vi "Format CSV.vi"(8 "error in (no error)":errorcluster, 9 "delimiter":string=",", 10 "CSV File Input":path, 11 "Original CSV Format":enum16{"Format A", "Format B"}(ring)) -> (0 "error out":errorcluster, 1 "Parcel Length":i32[](array[numeric]), 2 "All Terminal Data":T1(array[cluster]))   [LabVIEW 2017] (continued)
"32:42.2", "32:42.2", "32:42.3", "32:42.3", "32:42.3", "32:42.4", "32:42.4", "32:42.4", "32:42.5", "32:42.5", "32:42.5", "32:42.6", "32:42.6", "32:42.6", "32:42.7", "32:42.7", "32:42.7", "32:42.8", "32:42.8", "32:42.8", "32:42.9", "32:42.9", "32:42.9", "32:43.0", "32:43.0", "32:43.0", "32:43.1", "32:43.1", "32:43.1", "32:43.2", "32:43.2", "32:43.2", "32:43.3", "32:43.3", "32:43.3", "32:43.4", "32:43.4", "32:43.4", "32:43.5", "32:43.5", "32:43.5", "32:43.6", "32:43.6", "32:43.6", "32:43.7", "32:43.7", "32:43.7", "32:43.8", "32:43.8", "32:43.8", "32:43.9", "32:43.9", "32:43.9", "32:44.0", "32:44.0", "32:44.0", "32:44.1", "32:44.1", "32:44.1", "32:44.2", "32:44.2", "32:44.2", "32:44.3", "32:44.3", "32:44.3", "32:44.4", "32:44.4", "32:44.4", "32:44.5", "32:44.5", "32:44.5", "32:44.6", "32:44.6", "32:44.6", "32:44.7", "32:44.7", "32:44.7", "32:44.8", "32:44.8", "32:44.8", "32:44.9", "32:44.9", "32:44.9", "32:45.0", "32:45.0", "32:45.0", "32:45.1", "32:45.1", "32:45.1", "32:45.2", "32:45.2", "32:45.2", "32:45.3", "32:45.3", "32:45.3", "32:45.4", "32:45.4", "32:45.4", "32:45.5", "32:45.5", "32:45.5", "32:45.6", "32:45.6", "32:45.6", "32:45.7", "32:45.7", "32:45.7", "32:45.8", "32:45.8", "32:45.8", "32:45.9", "32:45.9", "32:45.9", "32:46.0", "32:46.0", "32:46.0", "32:46.1", "32:46.1", "32:46.1", "32:46.2", "32:46.2", "32:46.2", "32:46.3", "32:46.3", "32:46.3", "32:46.4", "32:46.4", "32:46.4", "32:46.5", "32:46.5", "32:46.5", "32:46.6", "32:46.6", "32:46.6", "32:46.7", "32:46.7", "32:46.7", "32:46.8", "32:46.8", "32:46.8", "32:46.9", "32:46.9", "32:46.9", "32:47.0", "32:47.0", "32:47.0", "32:47.1", "32:47.1", "32:47.1", "32:47.2", "32:47.2", "32:47.2", "32:47.3", "32:47.3", "32:47.3", "32:47.4", "32:47.4", "32:47.4", "32:47.5", "32:47.5", "32:47.5", "32:47.6", "32:47.6", "32:47.6", "32:47.7", "32:47.7", "32:47.7", "32:47.8", "32:47.8", "32:47.8", "32:47.9", "32:47.9", "32:47.9", "32:48.0", "32:48.0", "32:48.0", "32:48.1", "32:48.1", "32:48.1", "32:48.2", "32:48.2", "32:48.2", "32:48.3", "32:48.3", "32:48.3", "32:48.4", "32:48.4", "32:48.4", "32:48.5", "32:48.5", "32:48.5", "32:48.6", "32:48.6", "32:48.6", "32:48.7", "32:48.7", "32:48.7", "32:48.8", "32:48.8", "32:48.8", "32:48.9", "32:48.9", "32:48.9", "32:49.0", "32:49.0", "32:49.0", "32:49.1", "32:49.1", "32:49.1", "32:49.2", "32:49.2", "32:49.2", "32:49.3", "32:49.3", "32:49.3", "32:49.4", "32:49.4", "32:49.4", "32:49.5", "32:49.5", "32:49.5", "32:49.6", "32:49.6", "32:49.6", "32:49.7", "32:49.7", "32:49.7", "32:49.8", "32:49.8", "32:49.8", "32:49.9", "32:49.9", "32:49.9", "32:50.0", "32:50.0", "32:50.0", "32:50.1", "32:50.1", "32:50.1", "32:50.2", "32:50.2", "32:50.2", "32:50.3", "32:50.3", "32:50.3", "32:50.4", "32:50.4", "32:50.4", "32:50.5", "32:50.5", "32:50.5", "32:50.6", "32:50.6", "32:50.6", "32:50.7", "32:50.7", "32:50.7", "32:50.8", "32:50.8", "32:50.8", "32:50.9", "32:50.9", "32:50.9", "32:51.0", "32:51.0", "32:51.0", "32:51.1", "32:51.1", "32:51.1", "32:51.2", "32:51.2", "32:51.2", "32:51.3", "32:51.3", "32:51.3", "32:51.4", "32:51.4", "32:51.4", "32:51.5", "32:51.5", "32:51.5", "32:51.6", "32:51.6", "32:51.6", "32:51.7", "32:51.7", "32:51.7", "32:51.8", "32:51.8", "32:51.8", "32:51.9", "32:51.9", "32:51.9", "32:52.0", "32:52.0", "32:52.0", "32:52.1", "32:52.1", "32:52.1", "32:52.2", "32:52.2", "32:52.2", "32:52.3", "32:52.3", "32:52.3", "32:52.4", "32:52.4", "32:52.4", "32:52.5", "32:52.5", "32:52.5", "32:52.6", "32:52.6", "32:52.6", "32:52.7", "32:52.7", "32:52.7", "32:52.8", "32:52.8", "32:52.8", "32:52.9", "32:52.9", "32:52.9", "32:53.0", "32:53.0", "32:53.0", "32:53.1", "32:53.1", "32:53.1", "32:53.2", "32:53.2", "32:53.2", "32:53.3", "32:53.3", "32:53.3", "32:53.4", "32:53.4", "32:53.4", "32:53.5", "32:53.5", "32:53.5", "32:53.6", "32:53.6", "32:53.6", "32:53.7", "32:53.7", "32:53.7", "32:53.8", "32:53.8", "32:53.8", "32:53.9", "32:53.9", "32:53.9", "32:54.0", "32:54.0", "32:54.0", "32:54.1", "32:54.1", "32:54.1", "32:54.2", "32:54.2", "32:54.2", "32:54.3", "32:54.3", "32:54.3", "32:54.4", "32:54.4", "32:54.4", "32:54.5", "32:54.5", "32:54.5", "32:54.6", "32:54.6", "32:54.6", "32:54.7", "32:54.7", "32:54.7", "32:54.8", "32:54.8", "32:54.8", "32:54.9", "32:54.9", "32:54.9", "32:55.0", "32:55.0", "32:55.0", "32:55.1", "32:55.1", "32:55.1", "32:55.2", "32:55.2", "32:55.2", "32:55.3", "32:55.3", "32:55.3", "32:55.4", "32:55.4", "32:55.4", "32:55.5", "32:55.5", "32:55.5", "32:55.6", "32:55.6", "32:55.6", "32:55.7", "32:55.7", "32:55.7", "32:55.8", "32:55.8", "32:55.8", "32:55.9", "32:55.9", "32:55.9", "32:56.0", "32:56.0", "32:56.0", "32:56.1", "32:56.1", "32:56.1", "32:56.2", "32:56.2", "32:56.2", "32:56.3", "32:56.3", "32:56.3", "32:56.4", "32:56.4", "32:56.4", "32:56.5", "32:56.5", "32:56.5", "32:56.6", "32:56.6", "32:56.6", "32:56.7", "32:56.7", "32:56.7", "32:56.8", "32:56.8", "32:56.8", "32:56.9", "32:56.9", "32:56.9", "32:57.0", "32:57.0", "32:57.0", "32:57.1", "32:57.1", "32:57.1", "32:57.2", "32:57.2", "32:57.2", "32:57.3", "32:57.3", "32:57.3", "32:57.4", "32:57.4", "32:57.4", "32:57.5", "32:57.5", "32:57.5", "32:57.6", "32:57.6", "32:57.6", "32:57.7", "32:57.7", "32:57.7", "32:57.8", "32:57.8", "32:57.8", "32:57.9", "32:57.9", "32:57.9", "32:58.0", "32:58.0", "32:58.0", "32:58.1", "32:58.1", "32:58.1", "32:58.2", "32:58.2", "32:58.2", "32:58.3", "32:58.3", "32:58.3", "32:58.4", "32:58.4", "32:58.4", "32:58.5", "32:58.5", "32:58.5", "32:58.6", "32:58.6", "32:58.6", "32:58.7", "32:58.7", "32:58.7", "32:58.8", "32:58.8", "32:58.8", "32:58.9", "32:58.9", "32:58.9", "32:59.0", "32:59.0", "32:59.0", "32:59.1", "32:59.1", "32:59.1", "32:59.2", "32:59.2", "32:59.2", "32:59.3", "32:59.3", "32:59.3", "32:59.4", "32:59.4", "32:59.4", "32:59.5", "32:59.5", "32:59.5", "32:59.6", "32:59.6", "32:59.6", "32:59.7", "32:59.7", "32:59.7", "32:59.8", "32:59.8", "32:59.8", "32:59.9", "32:59.9", "32:59.9", "33:00.0", "33:00.0", "33:00.0", "33:00.1", "33:00.1", "33:00.1", "33:00.2", "33:00.2", "33:00.2", "33:00.3", "33:00.3", "33:00.3", "33:00.4", "33:00.4", "33:00.4", "33:00.5", "33:00.5", "33:00.5", "33:00.6", "33:00.6", "33:00.6", "33:00.7", "33:00.7", "33:00.7", "33:00.8", "33:00.8", "33:00.8", "33:00.9", "33:00.9", "33:00.9", "33:01.0", "33:01.0", "33:01.0", "33:01.1", "33:01.1", "33:01.1", "33:01.2", "33:01.2", "33:01.2", "33:01.3", "33:01.3", "33:01.3", "33:01.4", "33:01.4", "33:01.4", "33:01.5", "33:01.5", "33:01.5", "33:01.6", "33:01.6", "33:01.6", "33:01.7", "33:01.7", "33:01.7", "33:01.8", "33:01.8", "33:01.8", "33:01.9", "33:01.9", "33:01.9", "33:02.0", "33:02.0", "33:02.0", "33:02.1", "33:02.1", "33:02.1", "33:02.2", "33:02.2", "33:02.2", "33:02.3", "33:02.3", "33:02.3", "33:02.4", "33:02.4", "33:02.4", "33:02.5", "33:02.5", "33:02.5", "33:02.6", "33:02.6", "33:02.6", "33:02.7", "33:02.7", "33:02.7", "33:02.8", "33:02.8", "33:02.8", "33:02.9", "33:02.9", "33:02.9", "33:03.0", "33:03.0", "33:03.0", "33:03.1", "33:03.1", "33:03.1", "33:03.2", "33:03.2", "33:03.2", "33:03.3", "33:03.3", "33:03.3", "33:03.4", "33:03.4", "33:03.4", "33:03.5", "33:03.5", "33:03.5", "33:03.6", "33:03.6", "33:03.6", "33:03.7", "33:03.7", "33:03.7", "33:03.8", "33:03.8", "33:03.8", "33:03.9", "33:03.9", "33:03.9", "33:04.0", "33:04.0", "33:04.0", "33:04.1", "33:04.1", "33:04.1", "33:04.2", "33:04.2", "33:04.2", "33:04.3", "33:04.3", "33:04.3", "33:04.4", "33:04.4", "33:04.4", "33:04.5", "33:04.5", "33:04.5", "33:04.6", "33:04.6", "33:04.6", "33:04.7", "33:04.7", "33:04.7", "33:04.8", "33:04.8", "33:04.8", "33:04.9", "33:04.9", "33:04.9", "33:05.0", "33:05.0", "33:05.0", "33:05.1", "33:05.1", "33:05.1", "33:05.2", "33:05.2", "33:05.2", "33:05.3", "33:05.3", "33:05.3", "33:05.4", "33:05.4", "33:05.4", "33:05.5", "33:05.5", "33:05.5", "33:05.6", "33:05.6", "33:05.6", "33:05.7", "33:05.7", "33:05.7", "33:05.8", "33:05.8", "33:05.8", "33:05.9", "33:05.9", "33:05.9", "33:06.0", "33:06.0", "33:06.0", "33:06.1", "33:06.1", "33:06.1", "33:06.2", "33:06.2", "33:06.2", "33:06.3", "33:06.3", "33:06.3", "33:06.4", "33:06.4", "33:06.4", "33:06.5", "33:06.5", "33:06.5", "33:06.6", "33:06.6", "33:06.6", "33:06.7", "33:06.7", "33:06.7", "33:06.8", "33:06.8", "33:06.8", "33:06.9", "33:06.9", "33:06.9", "33:07.0", "33:07.0", "33:07.0", "33:07.1", "33:07.1", "33:07.1", "33:07.2", "33:07.2", "33:07.2", "33:07.3", "33:07.3", "33:07.3", "33:07.4", "33:07.4", "33:07.4", "33:07.5", "33:07.5", "33:07.5", "33:07.6", "33:07.6", "33:07.6", "33:07.7", "33:07.7", "33:07.7", "33:07.8", "33:07.8", "33:07.8", "33:07.9", "33:07.9", "33:07.9", "33:08.0", "33:08.0", "33:08.0", "33:08.1", "33:08.1", "33:08.1", "33:08.2", "33:08.2", "33:08.2", "33:08.3", "33:08.3", "33:08.3", "33:08.4", "33:08.4", "33:08.4", "33:08.5", "33:08.5", "33:08.5", "33:08.6", "33:08.6", "33:08.6", "33:08.7", "33:08.7", "33:08.7", "33:08.8", "33:08.8", "33:08.8", "33:08.9", "33:08.9", "33:08.9", "33:09.0", "33:09.0", "33:09.0", "33:09.1", "33:09.1", "33:09.1", "33:09.2", "33:09.2", "33:09.2", "33:09.3", "33:09.3", "33:09.3", "33:09.4", "33:09.4", "33:09.4", "33:09.5", "33:09.5", "33:09.5", "33:09.6", "33:09.6", "33:09.6", "33:09.7", "33:09.7", "33:09.7", "33:09.8", "33:09.8", "33:09.8", "33:09.9", "33:09.9", "33:09.9", "33:10.0", "33:10.0", "33:10.0", "33:10.1", "33:10.1", "33:10.1", "33:10.2", "33:10.2", "33:10.2", "33:10.3", "33:10.3", "33:10.3", "33:10.4", "33:10.4", "33:10.4", "33:10.5", "33:10.5", "33:10.5", "33:10.6", "33:10.6", "33:10.6", "33:10.7", "33:10.7", "33:10.7", "33:10.8", "33:10.8", "33:10.8", "33:10.9", "33:10.9", "33:10.9", "33:11.0", "33:11.0", "33:11.0", "33:11.1", "33:11.1", "33:11.1", "33:11.2", "33:11.2", "33:11.2", "33:11.3", "33:11.3", "33:11.3", "33:11.4", "33:11.4", "33:11.4", "33:11.5", "33:11.5", "33:11.5", "33:11.6", "33:11.6", "33:11.6", "33:11.7", "33:11.7", "33:11.7", "33:11.8", "33:11.8", "33:11.8", "33:11.9", "33:11.9", "33:11.9", "33:12.0", "33:12.0", "33:12.0", "33:12.1", "33:12.1", "33:12.1", "33:12.2", "33:12.2", "33:12.2", "33:12.3", "33:12.3", "33:12.3", "33:12.4", "33:12.4", "33:12.4", "33:12.5", "33:12.5", "33:12.5", "33:12.6", "33:12.6", "33:12.6", "33:12.7", "33:12.7", "33:12.7", "33:12.8", "33:12.8", "33:12.8", "33:12.9", "33:12.9", "33:12.9", "33:13.0", "33:13.0", "33:13.0", "33:13.1", "33:13.1", "33:13.1", "33:13.2", "33:13.2", "33:13.2", "33:13.3", "33:13.3", "33:13.3", "33:13.4", "33:13.4", "33:13.4", "33:13.5", "33:13.5", "33:13.5", "33:13.6", "33:13.6", "33:13.6", "33:13.7", "33:13.7", "33:13.7", "33:13.8", "33:13.8", "33:13.8", "33:13.9", "33:13.9", "33:13.9", "33:14.0", "33:14.0", "33:14.0", "33:14.1", "33:14.1", "33:14.1", "33:14.2", "33:14.2", "33:14.2", "33:14.3", "33:14.3", "33:14.3", "33:14.4", "33:14.4", "33:14.4", "33:14.5", "33:14.5", "33:14.5", "33:14.6", "33:14.6", "33:14.6", "33:14.7", "33:14.7", "33:14.7", "33:14.8", "33:14.8", "33:14.8", "33:14.9", "33:14.9", "33:14.9", "33:15.0", "33:15.0", "33:15.0", "33:15.1", "33:15.1", "33:15.1", "33:15.2", "33:15.2", "33:15.2", "33:15.3", "33:15.3", "33:15.3", "33:15.4", "33:15.4", "33:15.4", "33:15.5", "33:15.5", "33:15.5", "33:15.6", "33:15.6", "33:15.6", "33:15.7", "33:15.7", "33:15.7", "33:15.8", "33:15.8", "33:15.8", "33:15.9", "33:15.9", "33:15.9", "33:16.0", "33:16.0", "33:16.0", "33:16.1", "33:16.1", "33:16.1", "33:16.2", "33:16.2", "33:16.2", "33:16.3", "33:16.3", "33:16.3", "33:16.4", "33:16.4", "33:16.4", "33:16.5", "33:16.5", "33:16.5", "33:16.6", "33:16.6", "33:16.6", "33:16.7", "33:16.7", "33:16.7", "33:16.8", "33:16.8", "33:16.8", "33:16.9", "33:16.9", "33:16.9", "33:17.0", "33:17.0", "33:17.0", "33:17.1", "33:17.1", "33:17.1", "33:17.2", "33:17.2", "33:17.2", "33:17.3", "33:17.3", "33:17.3", "33:17.4", "33:17.4", "33:17.4", "33:17.5", "33:17.5", "33:17.5", "33:17.6", "33:17.6", "33:17.6", "33:17.7", "33:17.7", "33:17.7", "33:17.8", "33:17.8", "33:17.8", "33:17.9", "33:17.9", "33:17.9", "33:18.0", "33:18.0", "33:18.0", "33:18.1", "33:18.1", "33:18.1", "33:18.2", "33:18.2", "33:18.2", "33:18.3", "33:18.3", "33:18.3", "33:18.4", "33:18.4", "33:18.4", "33:18.5", "33:18.5", "33:18.5", "33:18.6", "33:18.6", "33:18.6", "33:18.7", "33:18.7", "33:18.7", "33:18.8", "33:18.8", "33:18.8", "33:18.9", "33:18.9", "33:18.9", "33:19.0", "33:19.0", "33:19.0", "33:19.1", "33:19.1", "33:19.1", "33:19.2", "33:19.2", "33:19.2", "33:19.3", "33:19.3", "33:19.3", "33:19.4", "33:19.4", "33:19.4", "33:19.5", "33:19.5", "33:19.5", "33:19.6", "33:19.6", "33:19.6", "33:19.7", "33:19.7", "33:19.7", "33:19.8", "33:19.8", "33:19.8", "33:19.9", "33:19.9", "33:19.9", "33:20.0", "33:20.0", "33:20.0", "33:20.1", "33:20.1", "33:20.1", "33:20.2", "33:20.2", "33:20.2", "33:20.3", "33:20.3", "33:20.3", "33:20.4", "33:20.4", "33:20.4", "33:20.5", "33:20.5", "33:20.5", "33:20.6", "33:20.6", "33:20.6", "33:20.7", "33:20.7", "33:20.7", "33:20.8", "33:20.8", "33:20.8", "33:20.9", "33:20.9", "33:20.9", "33:21.0", "33:21.0", "33:21.0", "33:21.1", "33:21.1", "33:21.1", "33:21.2", "33:21.2", "33:21.2", "33:21.3", "33:21.3", "33:21.3", "33:21.4", "33:21.4", "33:21.4", "33:21.5", "33:21.5", "33:21.5", "33:21.6", "33:21.6", "33:21.6", "33:21.7", "33:21.7", "33:21.7", "33:21.8", "33:21.8", "33:21.8", "33:21.9", "33:21.9", "33:21.9", "33:22.0", "33:22.0", "33:22.0", "33:22.1", "33:22.1", "33:22.1", "33:22.2", "33:22.2", "33:22.2", "33:22.3", "33:22.3", "33:22.3", "33:22.4", "33:22.4", "33:22.4", "33:22.5", "33:22.5", "33:22.5", "33:22.6", "33:22.6", "33:22.6", "33:22.7", "33:22.7", "33:22.7", "33:22.8", "33:22.8", "33:22.8", "33:22.9", "33:22.9", "33:22.9", "33:23.0", "33:23.0", "33:23.0", "33:23.1", "33:23.1", "33:23.1", "33:23.2", "33:23.2", "33:23.2", "33:23.3", "33:23.3", "33:23.3", "33:23.4", "33:23.4", "33:23.4", "33:23.5", "33:23.5", "33:23.5", "33:23.6", "33:23.6", "33:23.6", "33:23.7", "33:23.7", "33:23.7", "33:23.8", "33:23.8", "33:23.8", "33:23.9", "33:23.9", "33:23.9", "33:24.0", "33:24.0", "33:24.0", "33:24.1", "33:24.1", "33:24.1", "33:24.2", "33:24.2", "33:24.2", "33:24.3", "33:24.3", "33:24.3", "33:24.4", "33:24.4", "33:24.4", "33:24.5", "33:24.5", "33:24.5", "33:24.6", "33:24.6", "33:24.6", "33:24.7", "33:24.7", "33:24.7", "33:24.8", "33:24.8", "33:24.8", "33:24.9", "33:24.9", "33:24.9", "33:25.0", "33:25.0", "33:25.0", "33:25.1", "33:25.1", "33:25.1", "33:25.2", "33:25.2", "33:25.2", "33:25.3", "33:25.3", "33:25.3", "33:25.4", "33:25.4", "33:25.4", "33:25.5", "33:25.5", "33:25.5", "33:25.6", "33:25.6", "33:25.6", "33:25.7", "33:25.7", "33:25.7", "33:25.8", "33:25.8", "33:25.8", "33:25.9", "33:25.9", "33:25.9", "33:26.0", "33:26.0", "33:26.0", "33:26.1", "33:26.1", "33:26.1", "33:26.2", "33:26.2", "33:26.2", "33:26.3", "33:26.3", "33:26.3", "33:26.4", "33:26.4", "33:26.4", "33:26.5", "33:26.5", "33:26.5", "33:26.6", "33:26.6", "33:26.6", "33:26.7", "33:26.7", "33:26.7", "33:26.8", "33:26.8", "33:26.8", "33:26.9", "33:26.9", "33:26.9", "33:27.0", "33:27.0", "33:27.0", "33:27.1", "33:27.1", "33:27.1", "33:27.2", "33:27.2", "33:27.2", "33:27.3", "33:27.3", "33:27.3", "33:27.4", "33:27.4", "33:27.4", "33:27.5", "33:27.5", "33:27.5", "33:27.6", "33:27.6", "33:27.6", "33:27.7", "33:27.7", "33:27.7", "33:27.8", "33:27.8", "33:27.8", "33:27.9", "33:27.9", "33:27.9", "33:28.0", "33:28.0", "33:28.0", "33:28.1", "33:28.1", "33:28.1", "33:28.2", "33:28.2", "33:28.2", "33:28.3", "33:28.3", "33:28.3", "33:28.4", "33:28.4", "33:28.4", "33:28.5", "33:28.5", "33:28.5", "33:28.6", "33:28.6", "33:28.6", "33:28.7", "33:28.7", "33:28.7", "33:28.8", "33:28.8", "33:28.8", "33:28.9", "33:28.9", "33:28.9", "33:29.0", "33:29.0", "33:29.0", "33:29.1", "33:29.1", "33:29.1", "33:29.2", "33:29.2", "33:29.2", "33:29.3", "33:29.3", "33:29.3", "33:29.4", "33:29.4", "33:29.4", "33:29.5", "33:29.5", "33:29.5", "33:29.6", "33:29.6", "33:29.6", "33:29.7", "33:29.7", "33:29.7", "33:29.8", "33:29.8", "33:29.8", "33:29.9", "33:29.9", "33:29.9", "33:30.0", "33:30.0", "33:30.0", "33:30.1", "33:30.1", "33:30.1", "33:30.2", "33:30.2", "33:30.2", "33:30.3", "33:30.3", "33:30.3", "33:30.4", "33:30.4", "33:30.4", "33:30.5", "33:30.5", "33:30.5", "33:30.6", "33:30.6", "33:30.6", "33:30.7", "33:30.7", "33:30.7", "33:30.8", "33:30.8", "33:30.8", "33:30.9", "33:30.9", "33:30.9", "33:31.0", "33:31.0", "33:31.0", "33:31.1", "33:31.1", "33:31.1", "33:31.2", "33:31.2", "33:31.2", "33:31.3", "33:31.3", "33:31.3", "33:31.4", "33:31.4", "33:31.4", "33:31.5", "33:31.5", "33:31.5", "33:31.6", "33:31.6", "33:31.6", "33:31.7", "33:31.7", "33:31.7", "33:31.8", "33:31.8", "33:31.8", "33:31.9", "33:31.9", "33:31.9", "33:32.0", "33:32.0", "33:32.0", "33:32.1", "33:32.1", "33:32.1", "33:32.2", "33:32.2", "33:32.2", "33:32.3", "33:32.3", "33:32.3", "33:32.4", "33:32.4", "33:32.4", "33:32.5", "33:32.5", "33:32.5", "33:32.6", "33:32.6", "33:32.6", "33:32.7", "33:32.7", "33:32.7", "33:32.8", "33:32.8", "33:32.8", "33:32.9", "33:32.9", "33:32.9", "33:33.0", "33:33.0", "33:33.0", "33:33.1", "33:33.1", "33:33.1", "33:33.2", "33:33.2", "33:33.2", "33:33.3", "33:33.3", "33:33.3", "33:33.4", "33:33.4", "33:33.4", "33:33.5", "33:33.5", "33:33.5", "33:33.6", "33:33.6", "33:33.6", "33:33.7", "33:33.7", "33:33.7", "33:33.8", "33:33.8", "33:33.8", "33:33.9", "33:33.9", "33:33.9", "33:34.0", "33:34.0", "33:34.0", "33:34.1", "33:34.1", "33:34.1", "33:34.2", "33:34.2", "33:34.2", "33:34.3", "33:34.3", "33:34.3", "33:34.4", "33:34.4", "33:34.4", "33:34.5", "33:34.5", "33:34.5", "33:34.6", "33:34.6", "33:34.6", "33:34.7", "33:34.7", "33:34.7", "33:34.8", "33:34.8", "33:34.8", "33:34.9", "33:34.9", "33:34.9", "33:35.0", "33:35.0", "33:35.0", "33:35.1", "33:35.1", "33:35.1", "33:35.2", "33:35.2", "33:35.2", "33:35.3", "33:35.3", "33:35.3", "33:35.4", "33:35.4", "33:35.4", "33:35.5", "33:35.5", "33:35.5", "33:35.6", "33:35.6", "33:35.6", "33:35.7", "33:35.7", "33:35.7", "33:35.8", "33:35.8", "33:35.8", "33:35.9", "33:35.9", "33:35.9", "33:36.0", "33:36.0", "33:36.0", "33:36.1", "33:36.1", "33:36.1", "33:36.2", "33:36.2", "33:36.2", "33:36.3", "33:36.3", "33:36.3", "33:36.4", "33:36.4", "33:36.4", "33:36.5", "33:36.5", "33:36.5", "33:36.6", "33:36.6", "33:36.6", "33:36.7", "33:36.7", "33:36.7", "33:36.8", "33:36.8", "33:36.8", "33:36.9", "33:36.9", "33:36.9", "33:37.0", "33:37.0", "33:37.0", "33:37.1", "33:37.1", "33:37.1", "33:37.2", "33:37.2", "33:37.2", "33:37.3", "33:37.3", "33:37.3", "33:37.4", "33:37.4", "33:37.4", "33:37.5", "33:37.5", "33:37.5", "33:37.6", "33:37.6", "33:37.6", "33:37.7", "33:37.7", "33:37.7", "33:37.8", "33:37.8", "33:37.8", "33:37.9", "33:37.9", "33:37.9", "33:38.0", "33:38.0", "33:38.0", "33:38.1", "33:38.1", "33:38.1", "33:38.2", "33:38.2", "33:38.2", "33:38.3", "33:38.3", "33:38.3", "33:38.4", "33:38.4", "33:38.4", "33:38.5", "33:38.5", "33:38.5", "33:38.6", "33:38.6", "33:38.6", "33:38.7", "33:38.7", "33:38.7", "33:38.8", "33:38.8", "33:38.8", "33:38.9", "33:38.9", "33:38.9", "33:39.0", "33:39.0", "33:39.0", "33:39.1", "33:39.1", "33:39.1", "33:39.2", "33:39.2", "33:39.2", "33:39.3", "33:39.3", "33:39.3", "33:39.4", "33:39.4", "33:39.4", "33:39.5", "33:39.5", "33:39.5", "33:39.6", "33:39.6", "33:39.6", "33:39.7", "33:39.7", "33:39.7", "33:39.8", "33:39.8", "33:39.8", "33:39.9", "33:39.9", "33:39.9", "33:40.0", "33:40.0", "33:40.0", "33:40.1", "33:40.1", "33:40.1", "33:40.2", "33:40.2", "33:40.2", "33:40.3", "33:40.3", "33:40.3", "33:40.4", "33:40.4", "33:40.4", "33:40.5", "33:40.5", "33:40.5", "33:40.6", "33:40.6", "33:40.6", "33:40.7", "33:40.7", "33:40.7", "33:40.8", "33:40.8", "33:40.8", "33:40.9", "33:40.9", "33:40.9", "33:41.0", "33:41.0", "33:41.0", "33:41.1", "33:41.1", "33:41.1", "33:41.2", "33:41.2", "33:41.2", "33:41.3", "33:41.3", "33:41.3", "33:41.4", "33:41.4", "33:41.4", "33:41.5", "33:41.5", "33:41.5", "33:41.6", "33:41.6", "33:41.6", "33:41.7", "33:41.7", "33:41.7", "33:41.8", "33:41.8", "33:41.8", "33:41.9", "33:41.9", "33:41.9", "33:42.0", "33:42.0", "33:42.0", "33:42.1", "33:42.1", "33:42.1", "33:42.2", "33:42.2", "33:42.2", "33:42.3", "33:42.3", "33:42.3", "33:42.4", "33:42.4", "33:42.4", "33:42.5", "33:42.5", "33:42.5", "33:42.6", "33:42.6", "33:42.6", "33:42.7", "33:42.7", "33:42.7", "33:42.8", "33:42.8", "33:42.8", "33:42.9", "33:42.9", "33:42.9", "33:43.0", "33:43.0", "33:43.0", "33:43.1", "33:43.1", "33:43.1", "33:43.2", "33:43.2", "33:43.2", "33:43.3", "33:43.3", "33:43.3", "33:43.4", "33:43.4", "33:43.4", "33:43.5", "33:43.5", "33:43.5", "33:43.6", "33:43.6", "33:43.6", "33:43.7", "33:43.7", "33:43.7", "33:43.8", "33:43.8", "33:43.8", "33:43.9", "33:43.9", "33:43.9", "33:44.0", "33:44.0", "33:44.0", "33:44.1", "33:44.1", "33:44.1", "33:44.2", "33:44.2", "33:44.2", "33:44.3", "33:44.3", "33:44.3", "33:44.4", "33:44.4", "33:44.4", "33:44.5", "33:44.5", "33:44.5", "33:44.6", "33:44.6", "33:44.6", "33:44.7", "33:44.7", "33:44.7", "33:44.8", "33:44.8", "33:44.8", "33:44.9", "33:44.9", "33:44.9", "33:45.0", "33:45.0", "33:45.0", "33:45.1", "33:45.1", "33:45.1", "33:45.2", "33:45.2", "33:45.2", "33:45.3", "33:45.3", "33:45.3", "33:45.4", "33:45.4", "33:45.4", "33:45.5", "33:45.5", "33:45.5", "33:45.6", "33:45.6", "33:45.6", "33:45.7", "33:45.7", "33:45.7", "33:45.8", "33:45.8", "33:45.8", "33:45.9", "33:45.9", "33:45.9", "33:46.0", "33:46.0", "33:46.0", "33:46.1", "33:46.1", "33:46.1", "33:46.2", "33:46.2", "33:46.2", "33:46.3", "33:46.3", "33:46.3", "33:46.4", "33:46.4", "33:46.4", "33:46.5", "33:46.5", "33:46.5", "33:46.6", "33:46.6", "33:46.6", "33:46.7", "33:46.7", "33:46.7", "33:46.8", "33:46.8", "33:46.8", "33:46.9", "33:46.9", "33:46.9", "33:47.0", "33:47.0", "33:47.0", "33:47.1", "33:47.1", "33:47.1", "33:47.2", "33:47.2", "33:47.2", "33:47.3", "33:47.3", "33:47.3", "33:47.4", "33:47.4", "33:47.4", "33:47.5", "33:47.5", "33:47.5", "33:47.6", "33:47.6", "33:47.6", "33:47.7", "33:47.7", "33:47.7", "33:47.8", "33:47.8", "33:47.8", "33:47.9", "33:47.9", "33:47.9", "33:48.0", "33:48.0", "33:48.0", "33:48.1", "33:48.1", "33:48.1", "33:48.2", "33:48.2", "33:48.2", "33:48.3", "33:48.3", "33:48.3", "33:48.4", "33:48.4", "33:48.4", "33:48.5", "33:48.5", "33:48.5", "33:48.6", "33:48.6", "33:48.6", "33:48.7", "33:48.7", "33:48.7", "33:48.8", "33:48.8", "33:48.8", "33:48.9", "33:48.9", "33:48.9", "33:49.0", "33:49.0", "33:49.0", "33:49.1", "33:49.1", "33:49.1", "33:49.2", "33:49.2", "33:49.2", "33:49.3", "33:49.3", "33:49.3", "33:49.4", "33:49.4", "33:49.4", "33:49.5", "33:49.5", "33:49.5", "33:49.6", "33:49.6", "33:49.6", "33:49.7", "33:49.7", "33:49.7", "33:49.8", "33:49.8", "33:49.8", "33:49.9", "33:49.9", "33:49.9", "33:50.0", "33:50.0", "33:50.0", "33:50.1", "33:50.1", "33:50.1", "33:50.2", "33:50.2", "33:50.2", "33:50.3", "33:50.3", "33:50.3", "33:50.4", "33:50.4", "33:50.4", "33:50.5", "33:50.5", "33:50.5", "33:50.6", "33:50.6", "33:50.6", "33:50.7", "33:50.7", "33:50.7", "33:50.8", "33:50.8", "33:50.8", "33:50.9", "33:50.9", "33:50.9", "33:51.0", "33:51.0", "33:51.0", "33:51.1", "33:51.1", "33:51.1", "33:51.2", "33:51.2", "33:51.2", "33:51.3", "33:51.3", "33:51.3", "33:51.4", "33:51.4", "33:51.4", "33:51.5", "33:51.5", "33:51.5", "33:51.6", "33:51.6", "33:51.6", "33:51.7", "33:51.7", "33:51.7", "33:51.8", "33:51.8", "33:51.8", "33:51.9", "33:51.9", "33:51.9", "33:52.0", "33:52.0", "33:52.0", "33:52.1", "33:52.1", "33:52.1", "33:52.2", "33:52.2", "33:52.2", "33:52.3", "33:52.3", "33:52.3", "33:52.4", "33:52.4", "33:52.4", "33:52.5", "33:52.5", "33:52.5", "33:52.6", "33:52.6", "33:52.6", "33:52.7", "33:52.7", "33:52.7", "33:52.8", "33:52.8", "33:52.8", "33:52.9", "33:52.9", "33:52.9", "33:53.0", "33:53.0", "33:53.0", "33:53.1", "33:53.1", "33:53.1", "33:53.2", "33:53.2", "33:53.2", "33:53.3", "33:53.3", "33:53.3", "33:53.4", "33:53.4", "33:53.4", "33:53.5", "33:53.5", "33:53.5", "33:53.6", "33:53.6", "33:53.6", "33:53.7", "33:53.7", "33:53.7", "33:53.8", "33:53.8", "33:53.8", "33:53.9", "33:53.9", "33:53.9", "33:54.0", "33:54.0", "33:54.0", "33:54.1", "33:54.1", "33:54.1", "33:54.2", "33:54.2", "33:54.2", "33:54.3", "33:54.3", "33:54.3", "33:54.4", "33:54.4", "33:54.4", "33:54.5", "33:54.5", "33:54.5", "33:54.6", "33:54.6", "33:54.6", "33:54.7", "33:54.7", "33:54.7", "33:54.8", "33:54.8", "33:54.8", "33:54.9", "33:54.9", "33:54.9", "33:55.0", "33:55.0", "33:55.0", "33:55.1", "33:55.1", "33:55.1", "33:55.2", "33:55.2", "33:55.2", "33:55.3", "33:55.3", "33:55.3", "33:55.4", "33:55.4", "33:55.4", "33:55.5", "33:55.5", "33:55.5", "33:55.6", "33:55.6", "33:55.6", "33:55.7", "33:55.7", "33:55.7", "33:55.8", "33:55.8", "33:55.8", "33:55.9", "33:55.9", "33:55.9", "33:56.0", "33:56.0", "33:56.0", "33:56.1", "33:56.1", "33:56.1", "33:56.2", "33:56.2", "33:56.2", "33:56.3", "33:56.3", "33:56.3", "33:56.4", "33:56.4", "33:56.4", "33:56.5", "33:56.5", "33:56.5", "33:56.6", "33:56.6", "33:56.6", "33:56.7", "33:56.7", "33:56.7", "33:56.8", "33:56.8", "33:56.8", "33:56.9", "33:56.9", "33:56.9", "33:57.0", "33:57.0", "33:57.0", "33:57.1", "33:57.1", "33:57.1", "33:57.2", "33:57.2", "33:57.2", "33:57.3", "33:57.3", "33:57.3", "33:57.4", "33:57.4", "33:57.4", "33:57.5", "33:57.5", "33:57.5", "33:57.6", "33:57.6", "33:57.6", "33:57.7", "33:57.7", "33:57.7", "33:57.8", "33:57.8", "33:57.8", "33:57.9", "33:57.9", "33:57.9", "33:58.0", "33:58.0", "33:58.0", "33:58.1", "33:58.1", "33:58.1", "33:58.2", "33:58.2", "33:58.2", "33:58.3", "33:58.3", "33:58.3", "33:58.4", "33:58.4", "33:58.4", "33:58.5", "33:58.5", "33:58.5", "33:58.6", "33:58.6", "33:58.6", "33:58.7", "33:58.7", "33:58.7", "33:58.8", "33:58.8", "33:58.8", "33:58.9", "33:58.9", "33:58.9", "33:59.0", "33:59.0", "33:59.0", "33:59.1", "33:59.1", "33:59.1", "33:59.2", "33:59.2", "33:59.2", "33:59.3", "33:59.3", "33:59.3", "33:59.4", "33:59.4", "33:59.4", "33:59.5", "33:59.5", "33:59.5", "33:59.6", "33:59.6", "33:59.6", "33:59.7", "33:59.7", "33:59.7", "33:59.8", "33:59.8", "33:59.8", "33:59.9", "33:59.9", "33:59.9", "34:00.0", "34:00.0", "34:00.0", "34:00.1", "34:00.1", "34:00.1", "34:00.2", "34:00.2", "34:00.2", "34:00.3", "34:00.3", "34:00.3", "34:00.4", "34:00.4", "34:00.4", "34:00.5", "34:00.5", "34:00.5", "34:00.6", "34:00.6", "34:00.6", "34:00.7", "34:00.7", "34:00.7", "34:00.8", "34:00.8", "34:00.8", "34:00.9", "34:00.9", "34:00.9", "34:01.0", "34:01.0", "34:01.0", "34:01.1", "34:01.1", "34:01.1", "34:01.2", "34:01.2", "34:01.2", "34:01.3", "34:01.3", "34:01.3", "34:01.4", "34:01.4", "34:01.4", "34:01.5", "34:01.5", "34:01.5", "34:01.6", "34:01.6", "34:01.6", "34:01.7", "34:01.7", "34:01.7", "34:01.8", "34:01.8", "34:01.8", "34:01.9", "34:01.9", "34:01.9", "34:02.0", "34:02.0", "34:02.0", "34:02.1", "34:02.1", "34:02.1", "34:02.2", "34:02.2", "34:02.2", "34:02.3", "34:02.3", "34:02.3", "34:02.4", "34:02.4", "34:02.4", "34:02.5", "34:02.5", "34:02.5", "34:02.6", "34:02.6", "34:02.6", "34:02.7", "34:02.7", "34:02.7", "34:02.8", "34:02.8", "34:02.8", "34:02.9", "34:02.9", "34:02.9", "34:03.0", "34:03.0", "34:03.0", "34:03.1", "34:03.1", "34:03.1", "34:03.2", "34:03.2", "34:03.2", "34:03.3", "34:03.3", "34:03.3", "34:03.4", "34:03.4", "34:03.4", "34:03.5", "34:03.5", "34:03.5", "34:03.6", "34:03.6", "34:03.6", "34:03.7", "34:03.7", "34:03.7", "34:03.8", "34:03.8", "34:03.8", "34:03.9", "34:03.9", "34:03.9", "34:04.0", "34:04.0", "34:04.0", "34:04.1", "34:04.1", "34:04.1", "34:04.2", "34:04.2", "34:04.2", "34:04.3", "34:04.3", "34:04.3", "34:04.4", "34:04.4", "34:04.4", "34:04.5", "34:04.5", "34:04.5", "34:04.6", "34:04.6", "34:04.6", "34:04.7", "34:04.7", "34:04.7", "34:04.8", "34:04.8", "34:04.8", "34:04.9", "34:04.9", "34:04.9", "34:05.0", "34:05.0", "34:05.0", "34:05.1", "34:05.1", "34:05.1", "34:05.2", "34:05.2", "34:05.2", "34:05.3", "34:05.3", "34:05.3", "34:05.4", "34:05.4", "34:05.4", "34:05.5", "34:05.5", "34:05.5", "34:05.6", "34:05.6", "34:05.6", "34:05.7", "34:05.7", "34:05.7", "34:05.8", "34:05.8", "34:05.8", "34:05.9", "34:05.9", "34:05.9", "34:06.0", "34:06.0", "34:06.0", "34:06.1", "34:06.1", "34:06.1", "34:06.2", "34:06.2", "34:06.2", "34:06.3", "34:06.3", "34:06.3", "34:06.4", "34:06.4", "34:06.4", "34:06.5", "34:06.5", "34:06.5", "34:06.6", "34:06.6", "34:06.6", "34:06.7", "34:06.7", "34:06.7", "34:06.8", "34:06.8", "34:06.8", "34:06.9", "34:06.9", "34:06.9", "34:07.0", "34:07.0", "34:07.0", "34:07.1", "34:07.1", "34:07.1", "34:07.2", "34:07.2", "34:07.2", "34:07.3", "34:07.3", "34:07.3", "34:07.4", "34:07.4", "34:07.4", "34:07.5", "34:07.5", "34:07.5", "34:07.6", "34:07.6", "34:07.6", "34:07.7", "34:07.7", "34:07.7", "34:07.8", "34:07.8", "34:07.8", "34:07.9", "34:07.9", "34:07.9", "34:08.0", "34:08.0", "34:08.0", "34:08.1", "34:08.1", "34:08.1", "34:08.2", "34:08.2", "34:08.2", "34:08.3", "34:08.3", "34:08.3", "34:08.4", "34:08.4", "34:08.4", "34:08.5", "34:08.5", "34:08.5", "34:08.6", "34:08.6", "34:08.6", "34:08.7", "34:08.7", "34:08.7", "34:08.8", "34:08.8", "34:08.8", "34:08.9", "34:08.9", "34:08.9", "34:09.0", "34:09.0", "34:09.0", "34:09.1", "34:09.1", "34:09.1", "34:09.2", "34:09.2", "34:09.2", "34:09.3", "34:09.3", "34:09.3", "34:09.4", "34:09.4", "34:09.4", "34:09.5", "34:09.5", "34:09.5", "34:09.6", "34:09.6", "34:09.6", "34:09.7", "34:09.7", "34:09.7", "34:09.8", "34:09.8", "34:09.8", "34:09.9", "34:09.9", "34:09.9", "34:10.0", "34:10.0", "34:10.0", "34:10.1", "34:10.1", "34:10.1", "34:10.2", "34:10.2", "34:10.2", "34:10.3", "34:10.3", "34:10.3", "34:10.4", "34:10.4", "34:10.4", "34:10.5", "34:10.5", "34:10.5", "34:10.6", "34:10.6", "34:10.6", "34:10.7", "34:10.7", "34:10.7", "34:10.8", "34:10.8", "34:10.8", "34:10.9", "34:10.9", "34:10.9", "34:11.0", "34:11.0", "34:11.0", "34:11.1", "34:11.1", "34:11.1", "34:11.2", "34:11.2", "34:11.2", "34:11.3", "34:11.3", "34:11.3", "34:11.4", "34:11.4", "34:11.4", "34:11.5", "34:11.5", "34:11.5", "34:11.6", "34:11.6", "34:11.6", "34:11.7", "34:11.7", "34:11.7", "34:11.8", "34:11.8", "34:11.8", "34:11.9", "34:11.9", "34:11.9", "34:12.0", "34:12.0", "34:12.0", "34:12.1", "34:12.1", "34:12.1", "34:12.2", "34:12.2", "34:12.2", "34:12.3", "34:12.3", "34:12.3", "34:12.4", "34:12.4", "34:12.4", "34:12.5", "34:12.5", "34:12.5", "34:12.6", "34:12.6", "34:12.6", "34:12.7", "34:12.7", "34:12.7", "34:12.8", "34:12.8", "34:12.8", "34:12.9", "34:12.9", "34:12.9", "34:13.0", "34:13.0", "34:13.0", "34:13.1", "34:13.1", "34:13.1", "34:13.2", "34:13.2", "34:13.2", "34:13.3", "34:13.3", "34:13.3", "34:13.4", "34:13.4", "34:13.4", "34:13.5", "34:13.5", "34:13.5", "34:13.6", "34:13.6", "34:13.6", "34:13.7", "34:13.7", "34:13.7", "34:13.8", "34:13.8", "34:13.8", "34:13.9", "34:13.9", "34:13.9", "34:14.0", "34:14.0", "34:14.0", "34:14.1", "34:14.1", "34:14.1", "34:14.2", "34:14.2", "34:14.2", "34:14.3", "34:14.3", "34:14.3", "34:14.4", "34:14.4", "34:14.4", "34:14.5", "34:14.5", "34:14.5", "34:14.6", "34:14.6", "34:14.6", "34:14.7", "34:14.7", "34:14.7", "34:14.8", "34:14.8", "34:14.8", "34:14.9", "34:14.9", "34:14.9", "34:15.0", "34:15.0", "34:15.0", "34:15.1", "34:15.1", "34:15.1", "34:15.2", "34:15.2", "34:15.2", "34:15.3", "34:15.3", "34:15.3", "34:15.4", "34:15.4", "34:15.4", "34:15.5", "34:15.5", "34:15.5", "34:15.6", "34:15.6", "34:15.6", "34:15.7", "34:15.7", "34:15.7", "34:15.8", "34:15.8", "34:15.8", "34:15.9", "34:15.9", "34:15.9", "34:16.0", "34:16.0", "34:16.0", "34:16.1", "34:16.1", "34:16.1", "34:16.2", "34:16.2", "34:16.2", "34:16.3", "34:16.3", "34:16.3", "34:16.4", "34:16.4", "34:16.4", "34:16.5", "34:16.5", "34:16.5", "34:16.6", "34:16.6", "34:16.6", "34:16.7", "34:16.7", "34:16.7", "34:16.8", "34:16.8", "34:16.8", "34:16.9", "34:16.9", "34:16.9", "34:17.0", "34:17.0", "34:17.0", "34:17.1", "34:17.1", "34:17.1", "34:17.2", "34:17.2", "34:17.2", "34:17.3", "34:17.3", "34:17.3", "34:17.4", "34:17.4", "34:17.4", "34:17.5", "34:17.5", "34:17.5", "34:17.6", "34:17.6", "34:17.6", "34:17.7", "34:17.7", "34:17.7", "34:17.8", "34:17.8", "34:17.8", "34:17.9", "34:17.9", "34:17.9", "34:18.0", "34:18.0", "34:18.0", "34:18.1", "34:18.1", "34:18.1", "34:18.2", "34:18.2", "34:18.2", "34:18.3", "34:18.3", "34:18.3", "34:18.4", "34:18.4", "34:18.4", "34:18.5", "34:18.5", "34:18.5", "34:18.6", "34:18.6", "34:18.6", "34:18.7", "34:18.7", "34:18.7", "34:18.8", "34:18.8", "34:18.8", "34:18.9", "34:18.9", "34:18.9", "34:19.0", "34:19.0", "34:19.0", "34:19.1", "34:19.1", "34:19.1", "34:19.2", "34:19.2", "34:19.2", "34:19.3", "34:19.3", "34:19.3", "34:19.4", "34:19.4", "34:19.4", "34:19.5", "34:19.5", "34:19.5", "34:19.6", "34:19.6", "34:19.6", "34:19.7", "34:19.7", "34:19.7", "34:19.8", "34:19.8", "34:19.8", "34:19.9", "34:19.9", "34:19.9", "34:20.0", "34:20.0", "34:20.0", "34:20.1", "34:20.1", "34:20.1", "34:20.2", "34:20.2", "34:20.2", "34:20.3", "34:20.3", "34:20.3", "34:20.4", "34:20.4", "34:20.4", "34:20.5", "34:20.5", "34:20.5", "34:20.6", "34:20.6", "34:20.6", "34:20.7", "34:20.7", "34:20.7", "34:20.8", "34:20.8", "34:20.8", "34:20.9", "34:20.9", "34:20.9", "34:21.0", "34:21.0", "34:21.0", "34:21.1", "34:21.1", "34:21.1", "34:21.2", "34:21.2", "34:21.2", "34:21.3", "34:21.3", "34:21.3", "34:21.4", "34:21.4", "34:21.4", "34:21.5", "34:21.5", "34:21.5", "34:21.6", "34:21.6", "34:21.6", "34:21.7", "34:21.7", "34:21.7", "34:21.8", "34:21.8", "34:21.8", "34:21.9", "34:21.9", "34:21.9", "34:22.0", "34:22.0", "34:22.0", "34:22.1", "34:22.1", "34:22.1", "34:22.2", "34:22.2", "34:22.2", "34:22.3", "34:22.3", "34:22.3", "34:22.4", "34:22.4", "34:22.4", "34:22.5", "34:22.5", "34:22.5", "34:22.6", "34:22.6", "34:22.6", "34:22.7", "34:22.7", "34:22.7", "34:22.8", "34:22.8", "34:22.8", "34:22.9", "34:22.9", "34:22.9", "34:23.0", "34:23.0", "34:23.0", "34:23.1", "34:23.1", "34:23.1", "34:23.2", "34:23.2", "34:23.2", "34:23.3", "34:23.3", "34:23.3", "34:23.4", "34:23.4", "34:23.4", "34:23.5", "34:23.5", "34:23.5", "34:23.6", "34:23.6", "34:23.6", "34:23.7", "34:23.7", "34:23.7", "34:23.8", "34:23.8", "34:23.8", "34:23.9", "34:23.9", "34:23.9", "34:24.0", "34:24.0", "34:24.0", "34:24.1", "34:24.1", "34:24.1", "34:24.2", "34:24.2", "34:24.2", "34:24.3", "34:24.3", "34:24.3", "34:24.4", "34:24.4", "34:24.4", "34:24.5", "34:24.5", "34:24.5", "34:24.6", "34:24.6", "34:24.6", "34:24.7", "34:24.7", "34:24.7", "34:24.8", "34:24.8", "34:24.8", "34:24.9", "34:24.9", "34:24.9", "34:25.0", "34:25.0", "34:25.0", "34:25.1", "34:25.1", "34:25.1", "34:25.2", "34:25.2", "34:25.2", "34:25.3", "34:25.3", "34:25.3", "34:25.4", "34:25.4", "34:25.4", "34:25.5", "34:25.5", "34:25.5", "34:25.6", "34:25.6", "34:25.6", "34:25.7", "34:25.7", "34:25.7", "34:25.8", "34:25.8", "34:25.8", "34:25.9", "34:25.9", "34:25.9", "34:26.0", "34:26.0", "34:26.0", "34:26.1", "34:26.1", "34:26.1", "34:26.2", "34:26.2", "34:26.2", "34:26.3", "34:26.3", "34:26.3", "34:26.4", "34:26.4", "34:26.4", "34:26.5", "34:26.5", "34:26.5", "34:26.6", "34:26.6", "34:26.6", "34:26.7", "34:26.7", "34:26.7", "34:26.8", "34:26.8", "34:26.8", "34:26.9", "34:26.9", "34:26.9", "34:27.0", "34:27.0", "34:27.0", "34:27.1", "34:27.1", "34:27.1", "34:27.2", "34:27.2", "34:27.2", "34:27.3", "34:27.3", "34:27.3", "34:27.4", "34:27.4", "34:27.4", "34:27.5", "34:27.5", "34:27.5", "34:27.6", "34:27.6", "34:27.6", "34:27.7", "34:27.7", "34:27.7", "34:27.8", "34:27.8", "34:27.8", "34:27.9", "34:27.9", "34:27.9", "34:28.0", "34:28.0", "34:28.0", "34:28.1", "34:28.1", "34:28.1", "34:28.2", "34:28.2", "34:28.2", "34:28.3", "34:28.3", "34:28.3", "34:28.4", "34:28.4", "34:28.4", "34:28.5", "34:28.5", "34:28.5", "34:28.6", "34:28.6", "34:28.6", "34:28.7", "34:28.7", "34:28.7", "34:28.8", "34:28.8", "34:28.8", "34:28.9", "34:28.9", "34:28.9", "34:29.0", "34:29.0", "34:29.0", "34:29.1", "34:29.1", "34:29.1", "34:29.2", "34:29.2", "34:29.2", "34:29.3", "34:29.3", "34:29.3", "34:29.4", "34:29.4", "34:29.4", "34:29.5", "34:29.5", "34:29.5", "34:29.6", "34:29.6", "34:29.6", "34:29.7", "34:29.7", "34:29.7", "34:29.8", "34:29.8", "34:29.8", "34:29.9", "34:29.9", "34:29.9", "34:30.0", "34:30.0", "34:30.0", "34:30.1", "34:30.1", "34:30.1", "34:30.2", "34:30.2", "34:30.2", "34:30.3", "34:30.3", "34:30.3", "34:30.4", "34:30.4", "34:30.4", "34:30.5", "34:30.5", "34:30.5", "34:30.6", "34:30.6", "34:30.6", "34:30.7", "34:30.7", "34:30.7", "34:30.8", "34:30.8", "34:30.8", "34:30.9", "34:30.9", "34:30.9", "34:31.0", "34:31.0", "34:31.0", "34:31.1", "34:31.1", "34:31.1", "34:31.2", "34:31.2", "34:31.2", "34:31.3", "34:31.3", "34:31.3", "34:31.4", "34:31.4", "34:31.4", "34:31.5", "34:31.5", "34:31.5", "34:31.6", "34:31.6", "34:31.6", "34:31.7", "34:31.7", "34:31.7", "34:31.8", "34:31.8", "34:31.8", "34:31.9", "34:31.9", "34:31.9", "34:32.0", "34:32.0", "34:32.0", "34:32.1", "34:32.1", "34:32.1", "34:32.2", "34:32.2", "34:32.2", "34:32.3", "34:32.3", "34:32.3", "34:32.4", "34:32.4", "34:32.4", "34:32.5", "34:32.5", "34:32.5", "34:32.6", "34:32.6", "34:32.6", "34:32.7", "34:32.7", "34:32.7", "34:32.8", "34:32.8", "34:32.8", "34:32.9", "34:32.9", "34:32.9", "34:33.0", "34:33.0", "34:33.0", "34:33.1", "34:33.1", "34:33.1", "34:33.2", "34:33.2", "34:33.2", "34:33.3", "34:33.3", "34:33.3", "34:33.4", "34:33.4", "34:33.4", "34:33.5", "34:33.5", "34:33.5", "34:33.6", "34:33.6", "34:33.6", "34:33.7", "34:33.7", "34:33.7", "34:33.8", "34:33.8", "34:33.8", "34:33.9", "34:33.9", "34:33.9", "34:34.0", "34:34.0", "34:34.0", "34:34.1", "34:34.1", "34:34.1", "34:34.2", "34:34.2", "34:34.2", "34:34.3", "34:34.3", "34:34.3", "34:34.4", "34:34.4", "34:34.4", "34:34.5", "34:34.5", "34:34.5", "34:34.6", "34:34.6", "34:34.6", "34:34.7", "34:34.7", "34:34.7", "34:34.8", "34:34.8", "34:34.8", "34:34.9", "34:34.9", "34:34.9", "34:35.0", "34:35.0", "34:35.0", "34:35.1", "34:35.1", "34:35.1", "34:35.2", "34:35.2", "34:35.2", "34:35.3", "34:35.3", "34:35.3", "34:35.4", "34:35.4", "34:35.4", "34:35.5", "34:35.5", "34:35.5", "34:35.6", "34:35.6", "34:35.6", "34:35.7", "34:35.7", "34:35.7", "34:35.8", "34:35.8", "34:35.8", "34:35.9", "34:35.9", "34:35.9", "34:36.0", "34:36.0", "34:36.0", "34:36.1", "34:36.1", "34:36.1", "34:36.2", "34:36.2", "34:36.2", "34:36.3", "34:36.3", "34:36.3", "34:36.4", "34:36.4", "34:36.4", "34:36.5", "34:36.5", "34:36.5", "34:36.6", "34:36.6", "34:36.6", "34:36.7", "34:36.7", "34:36.7", "34:36.8", "34:36.8", "34:36.8", "34:36.9", "34:36.9", "34:36.9", "34:37.0", "34:37.0", "34:37.0", "34:37.1", "34:37.1", "34:37.1", "34:37.2", "34:37.2", "34:37.2", "34:37.3", "34:37.3", "34:37.3", "34:37.4", "34:37.4", "34:37.4", "34:37.5", "34:37.5", "34:37.5", "34:37.6", "34:37.6", "34:37.6", "34:37.7", "34:37.7", "34:37.7", "34:37.8", "34:37.8", "34:37.8", "34:37.9", "34:37.9", "34:37.9", "34:38.0", "34:38.0", "34:38.0", "34:38.1", "34:38.1", "34:38.1", "34:38.2", "34:38.2", "34:38.2", "34:38.3", "34:38.3", "34:38.3", "34:38.4", "34:38.4", "34:38.4", "34:38.5", "34:38.5", "34:38.5", "34:38.6", "34:38.6", "34:38.6", "34:38.7", "34:38.7", "34:38.7", "34:38.8", "34:38.8", "34:38.8", "34:38.9", "34:38.9", "34:38.9", "34:39.0", "34:39.0", "34:39.0", "34:39.1", "34:39.1", "34:39.1", "34:39.2", "34:39.2", "34:39.2", "34:39.3", "34:39.3", "34:39.3", "34:39.4", "34:39.4", "34:39.4", "34:39.5", "34:39.5", "34:39.5", "34:39.6", "34:39.6", "34:39.6", "34:39.7", "34:39.7", "34:39.7", "34:39.8", "34:39.8", "34:39.8", "34:39.9", "34:39.9", "34:39.9", "34:40.0", "34:40.0", "34:40.0", "34:40.1", "34:40.1", "34:40.1", "34:40.2", "34:40.2", "34:40.2", "34:40.3", "34:40.3", "34:40.3", "34:40.4", "34:40.4", "34:40.4", "34:40.5", "34:40.5", "34:40.5", "34:40.6", "34:40.6", "34:40.6", "34:40.7", "34:40.7", "34:40.7", "34:40.8", "34:40.8", "34:40.8", "34:40.9", "34:40.9", "34:40.9", "34:41.0", "34:41.0", "34:41.0", "34:41.1", "34:41.1", "34:41.1", "34:41.2", "34:41.2", "34:41.2", "34:41.3", "34:41.3", "34:41.3", "34:41.4", "34:41.4", "34:41.4", "34:41.5", "34:41.5", "34:41.5", "34:41.6", "34:41.6", "34:41.6", "34:41.7", "34:41.7", "34:41.7", "34:41.8", "34:41.8", "34:41.8", "34:41.9", "34:41.9", "34:41.9", "34:42.0", "34:42.0", "34:42.0", "34:42.1", "34:42.1", "34:42.1", "34:42.2", "34:42.2", "34:42.2", "34:42.3", "34:42.3", "34:42.3", "34:42.4", "34:42.4", "34:42.4", "34:42.5", "34:42.5", "34:42.5", "34:42.6", "34:42.6", "34:42.6", "34:42.7", "34:42.7", "34:42.7", "34:42.8", "34:42.8", "34:42.8", "34:42.9", "34:42.9", "34:42.9", "34:43.0", "34:43.0", "34:43.0", "34:43.1", "34:43.1", "34:43.1", "34:43.2", "34:43.2", "34:43.2", "34:43.3", "34:43.3", "34:43.3", "34:43.4", 
